vi "Write Value Type.vi"(8 "error in (no error)":errorcluster, 10 "Value Type":string, 11 "DriverSetting in":refnum<class "DriverSetting.lvclass">) -> (0 "error out":errorcluster, 3 "DriverSetting out":refnum<class "DriverSetting.lvclass">)   [LabVIEW 2023, in "HAF.lvlib" / "DriverSetting.lvclass"]
doc: "Saves a new data type for the value of this Driver Setting. The data type must be in the list of valid data types otherwise an error is raised."
uses:
  DriverSetting.lvclass
  DriverSetting.lvclass/DriverSetting.ctl
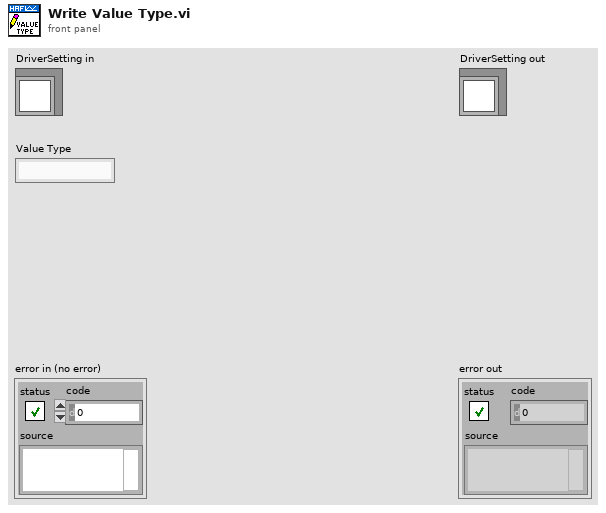
[diagram p1: front panel]
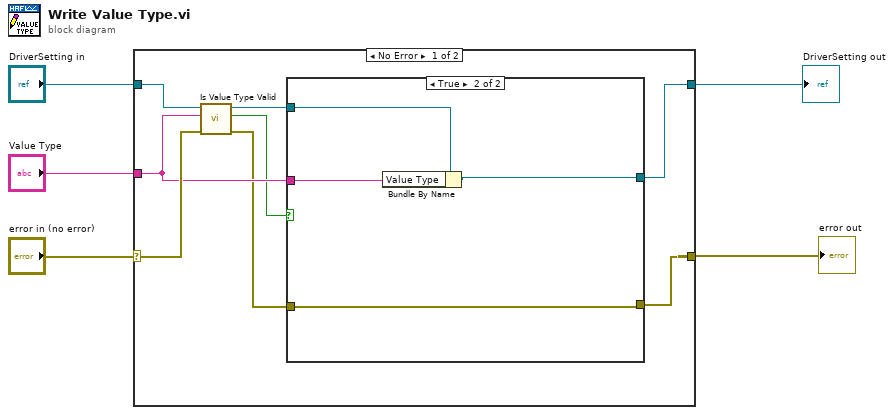
[diagram p0: block diagram]
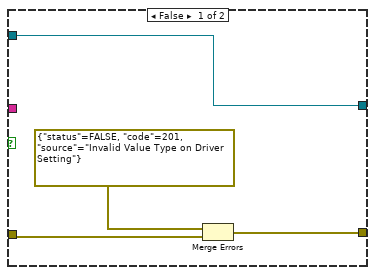
[diagram p2: hidden frame]
diagram:
  n1 = case shown="No Error" "error in (no error)" {
    selector: "error in (no error)" -> [w12 w22]
    tunnel: [w6 w22] -> w4
    tunnel: [w7 w23] -> w2
    tunnel: "DriverSetting in" -> [w13 w23]
    tunnel: "Value Type" -> [w11 _]
    frame No Error {
      n2 = call-dynamic "Is Value Type Valid.vi"("error in (no error)"=w12, "Value Type to Check"=w11, "DriverSetting in"=w13) -> ("error out"=w10:errorcluster, "Is Valid"=w8:bool, "DriverSetting out"=w9:refnum<class "DriverSetting.lvclass">)  [unwired: 6 in]
      n3 = case shown="True" w8 {
        tunnel: w11 -> [_ w21]
        tunnel: w10 -> [w16 w18]
        tunnel: w9 -> [w17 w20]
        tunnel: [w17 w19] -> w7
        tunnel: [w14 w18] -> w6
        frame False {
          n4 = Merge Errors(errorcluster {"status"=FALSE, "code"=201, "source"="Invalid Value Type on Driver Setting"} ("error in"), w16) -> (w14:errorcluster)
        }
        frame True {
          n5 = Bundle By Name(cluster=w20, "Value Type"=w21) -> (w19:refnum<class "DriverSetting.lvclass">)
        }
      }
    }
    frame Error {
    }
  }
  "error out" <- w4
  "DriverSetting out" <- w2
